vi "Module Cleanup.vi"(8 "error in (no error)":errorcluster, 11 "Telemetry Server in":refnum<class "Telemetry Server.lvclass">) -> (0 "error out":errorcluster, 3 "Telemetry Server out":refnum<class "Telemetry Server.lvclass">)   [LabVIEW 2020, in "VolatusTelemetry.lvlib" / "Telemetry Server.lvclass"]
uses:
  Telemetry Server.lvclass
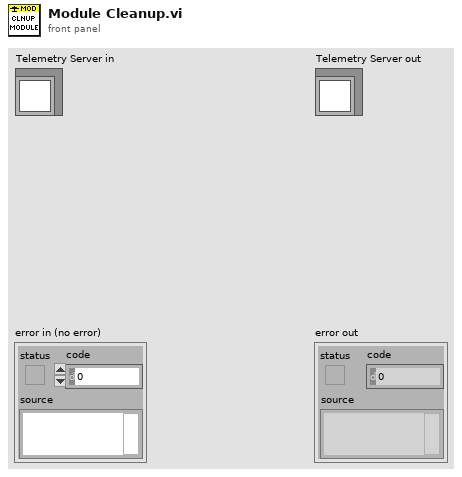
[diagram p1: front panel]
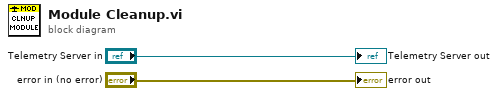
[diagram p0: block diagram]
diagram:
  "error out" <- "error in (no error)"
  "Telemetry Server out" <- "Telemetry Server in"
